vi "calibMagnetometersGetTransformations.vi"(8 "error in (no error)":errorcluster, 11 "pHandle":u32) -> (0 "error out":errorcluster, 1 "return type":i32, 2 "crossAxis":sgl[](array[numeric]), 3 "offset":sgl[](array[numeric]))   [LabVIEW 2011, in "sbgLabView.lvlib"]
uses:
  sbgLabView.lvlib
  sbgMatLab.dll
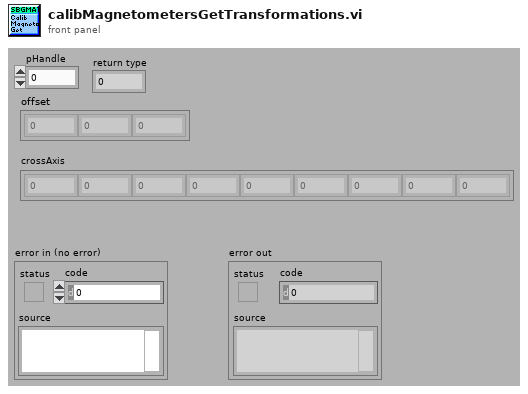
[diagram p1: front panel]
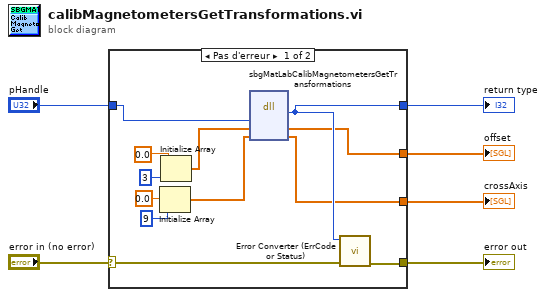
[diagram p0: block diagram]
diagram:
  n1 = case shown="Pas d'erreur" "error in (no error)" {
    selector: "error in (no error)" -> [w9 w19]
    tunnel: [w8 w19] -> w5
    tunnel: [w18 _] -> w4
    tunnel: "pHandle" -> [w17 _]
    tunnel: [w14 _] -> w2
    tunnel: [w10 _] -> w1
    frame No Error {
      n2 = Initialize Array(sgl 0.0 ("element"), 9 ("dimension size")) -> (w13:sgl[])
      n3 = Initialize Array(sgl 0.0 ("element"), 3 ("dimension size")) -> (w16:sgl[])
      n4 = dll-call lib="C:/SBG-Systems/remote/projects/software/projects/labviewExample/sbgLabView/sbgMatLab.*" fn="sbgMatLabCalibMagnetometersGetTransformations"("pHandle"=w17, "offset"=w16, "crossAxis"=w13) -> ("return type"=w18:i32, "offset"=w14:sgl[], "crossAxis"=w10:sgl[])  [unwired: 4 in, 2 out]
      n5 = call "Error Converter (ErrCode or Status).vi"("error in (no error)"=w9, "error code"=w18) -> ("error out"=w8:errorcluster)  [unwired: 9 in]
    }
    frame Error {
    }
  }
  "return type" <- w4
  "offset" <- w2
  "crossAxis" <- w1
  "error out" <- w5
